vi "Read WindowTime.vi"(8 "error in (no error)":errorcluster, 11 "AnalysisPluginsBase in":refnum<class "AnalysisPluginsBase.lvclass">) -> (0 "error out":errorcluster, 2 "WindowTime":dbl format="%.6g", 3 "AnalysisPluginsBase out":refnum<class "AnalysisPluginsBase.lvclass">)   [LabVIEW 2014, in "AnalysisPlugins.lvlib" / "AnalysisPluginsBase.lvclass"]
uses:
  AnalysisPluginsBase.lvclass
  AnalysisPluginsBase.lvclass/AnalysisPluginsBase.ctl
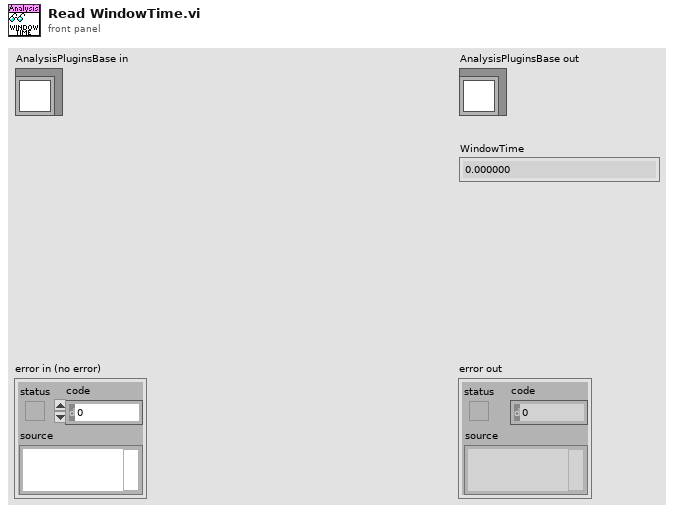
[diagram p1: front panel]
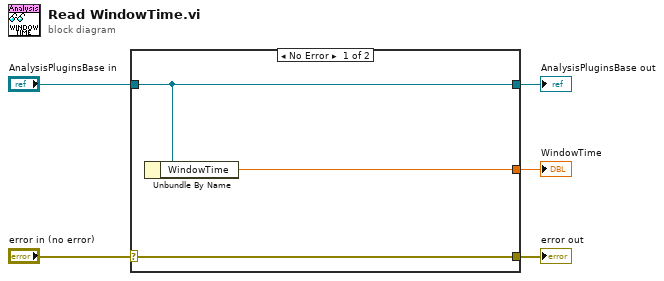
[diagram p0: block diagram]
diagram:
  n1 = case shown="No Error" "error in (no error)" {
    selector: "error in (no error)" -> [w8 w9]
    tunnel: [w8 w9] -> w4
    tunnel: [w7 w10] -> w2
    tunnel: "AnalysisPluginsBase in" -> [w7 w10]
    tunnel: [w6 _] -> w1
    frame No Error {
      n2 = Unbundle By Name(w7) -> ("WindowTime"=w6:dbl)
    }
    frame Error {
    }
  }
  "error out" <- w4
  "AnalysisPluginsBase out" <- w2
  "WindowTime" <- w1
